vi "GetWaveformData.vi"(8 "error in (no error)":errorcluster, 9 "Number of Samples":i32, 10 "Current Channel":string, 11 "Data Value Reference in":T3) -> (0 "error out":errorcluster, 3 "DataSet":T1)   [LabVIEW 2017, in "CmsTestPanel.lvlib"]
uses:
  <vilib>/addons/InsightCM/Devices/Shared/Cms/CmsTestPanel/CmsTestPanel.lvlib
  <vilib>/addons/InsightCM/Utilities/DataAccessors/controls/wfmSGL_DVR.ctl
  <vilib>/addons/InsightCM/MessageBus/Base/controls/DataSetByteData.ctl
  <vilib>/addons/InsightCM/MessageBus/Base/controls/KeyValuePair.ctl
  <vilib>/addons/InsightCM/Utilities/ChannelStatus/ChannelStatus.lvlib
  <vilib>/addons/InsightCM/Utilities/PropertyHelpers/PropertyHelpers.lvlib
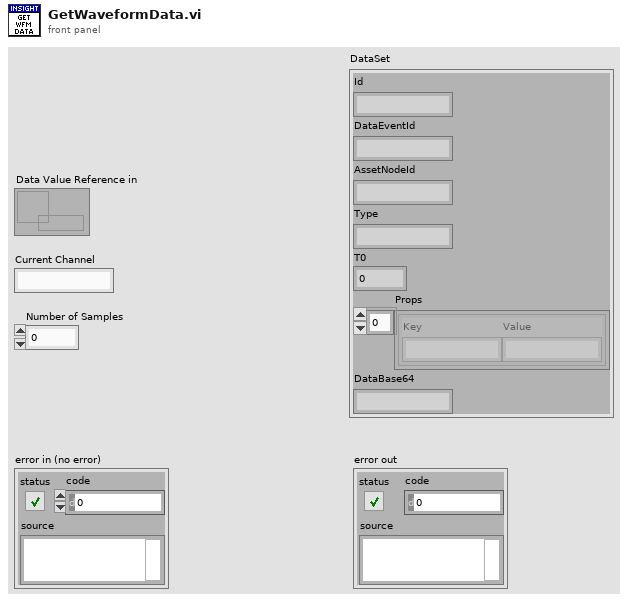
[diagram p1: front panel]
types:
  T1 = typedef "DataSetByteData.ctl" = cluster{"Id":string, "DataEventId":string, "AssetNodeId":string, "Type":string, "T0":i64, "Props":T2[], "DataBase64":string}
  T2 = typedef "KeyValuePair.ctl" = cluster{"Key":string, "Value":string}
  T3 = typedef "wfmSGL_DVR.ctl" = refnum<data-value>
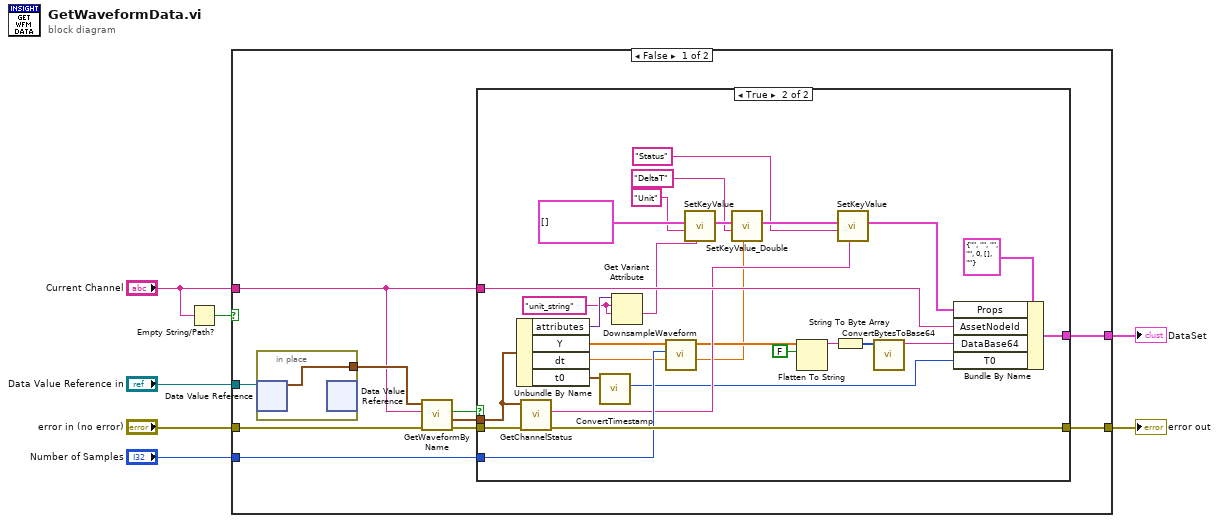
[diagram p0: block diagram]
diagram:
  n1 = Empty String/Path?(string/path="Current Channel") -> (empty?=w5:bool)
  n2 = case shown="False" w5 {
    tunnel: "Data Value Reference in" -> [w17 _]
    tunnel: [w13 w48] -> w3
    tunnel: "error in (no error)" -> [w16 w48]
    tunnel: "Current Channel" -> [w10 _]
    tunnel: "Number of Samples" -> [w9 _]
    tunnel: [w8 _] -> w1
    frame False {
      n3 = in-place {
        in-place-border: [w47] -> w15
        n4 = in-place-dvr #1(w17) -> (w47:waveform(sgl)[])  [unwired: 1 out]
        n5 = in-place-dvr #1() -> ()  [unwired: 1 in, 2 out]
      }
      n6 = call <vilib>:"GetWaveformByName.vi"("error in (no error)"=w16, "Channel Name"=w10, "Acq Waveforms"=w15) -> ("error out"=w12:errorcluster, "Waveform"=w11:waveform(sgl), "Found?"=w14:bool)  [unwired: 5 in, 1 out]
      n7 = case shown="True" w14 {
        tunnel: [w18 w45] -> w13
        tunnel: w12 -> [w18 w46]
        tunnel: w11 -> [_ w44]
        tunnel: w10 -> [_ w35]
        tunnel: w9 -> [_ w39]
        tunnel: [_ w28] -> w8
        frame False {
        }
        frame True {
          w41 = "unit_string" ("name")
          n8 = Unbundle By Name(w44) -> ("attributes"=w42:variant, "Y"=w40:sgl[], "dt"=w20:dbl, "t0"=w43:timestamp)
          n9 = call <vilib>:"GetChannelStatus.vi"("error in (no error)"=w46, "waveform in"=w44) -> ("error out"=w45:errorcluster, "channel status"=w29:string)  [unwired: 6 in, 2 out]
          n10 = call <vilib>:"ConvertTimestamp.vi"("Time Stamp"=w43) -> ("Timestamp out"=w27:i64)  [unwired: 10 in]
          n11 = Get Variant Attribute(Variant=w42, name=w41, default value (empty Variant)=w41) -> (value=w34:string)  [unwired: 1 in, 3 out]
          n12 = call <vilib>:"DownsampleWaveform.vi"("dt"=w20, "Number of Samples"=w39, "data"=w40) -> ("new dt"=w19:dbl, "values"=w23:sgl[])  [unwired: 7 in]
          n13 = call <vilib>:"SetKeyValue.vi"("value"=w34, "key"="Unit", "key value pairs"=T2[] []) -> ("key value pairs out"=w33:T2[])  [unwired: 8 in]
          n14 = call <vilib>:"SetKeyValue_Double.vi"("value"=w19, "key"="DeltaT", "key value pairs"=w33) -> ("key value pairs out"=w32:T2[])  [unwired: 8 in]
          n15 = Flatten To String(anything=w23, prepend array or string size? (T)=FALSE) -> (data string=w25:string)  [unwired: 2 in, 2 out]
          n16 = String To Byte Array(string=w25) -> (unsigned byte array=w22:u8[])
          n17 = call <vilib>:"SetKeyValue.vi"("value"=w29, "key"="Status", "key value pairs"=w32) -> ("key value pairs out"=w26:T2[])  [unwired: 8 in]
          n18 = call <vilib>:"ConvertBytesToBase64.vi"("U8 array"=w22) -> ("base64 encoded"=w21:string)  [unwired: 10 in]
          n19 = Bundle By Name(cluster=T1 {"Id"="", "DataEventId"="", "AssetNodeId"="", "Type"="", "T0"=0, "Props"=[], "DataBase64"=""} ("DataSet"), "Props"=w26, "AssetNodeId"=w35, "DataBase64"=w21, "T0"=w27) -> (w28:T1)
        }
      }
    }
    frame True {
    }
  }
  "error out" <- w3
  "DataSet" <- w1
